vi "ArdnoLoad.vi"(0 "LINX Resource":T1={"IO"=enum."Remote", "Interface"=enum."Serial", "LINX Device Config"={"Interface"=enum."Serial", "COM Port"="COM13", "TCP Configuration"={"IP Address"="", "Port"=0}, "Device Family"=1, "Device ID"=1, "Device Name"="myRIO-1900", "TCP Ref"=refnum, "Channels"={"DI"=[0, 1, 2, 3, 4, 5, 6, 7, 8, 9, 10, 11, 12, 13, 14, 15, 16, 17, 18, 19, 20, 21, 22, 23, 24, 25, 26, 27, 28, 29, 30, 31, 32, 33, 34, 35, 36, 37, 38, 39, 40, 41, 42, 43, 44, 45, 46], "DO"=[0, 1, 2, 3, 4, 5, 6, 7, 8, 9, 10, 11, 12, 13, 14, 15, 16, 17, 18, 19, 20, 21, 22, 23, 24, 25, 26, 27, 28, 29, 30, 31, 32, 33, 34, 35, 36, 37, 38, 39, 40, 41, 42, 43, 44, 45, 46], "AI"=[0, 1, 2, 3, 4, 5, 6, 7, 8, 9, 10, 11], "AO"=[], "PWM"=[3, 5, 6, 9, 10], "QE"=[], "UART"=[0, 1], "I2C 2"=[0], "SPI"=[0], "CAN"=[], "Servo"=[], "AI Ref (V)"=0.0, "AI Resolution (Bits)"=0, "AO Ref (V)"=0.0, "AO Resolution (Bits)"=0}}}, 1 "Single / Multiring?":u16(ring) items=["OneRing", "8-Ring"], 5 "Channel":u32, 7 "Ring":u16, 11 "error in (no error)":errorcluster, 12 "All Rings":bool) -> (4 "LINX Resource out":T1, 14 "ValveStates":bool[](array[boolean]), 15 "error out":errorcluster)   [LabVIEW 2018, in "Arduino.lvlib"]
uses:
  Arduino.lvlib
  <vilib>/MakerHub/LINX/Private/Type Defs/LINX Ref.ctl
  <vilib>/MakerHub/LINX/Private/Type Defs/Platform.ctl
  <vilib>/MakerHub/LINX/Private/Type Defs/Interface.ctl
  <vilib>/MakerHub/LINX/Private/Device/Type Defs/LINX Device Config.ctl
  <vilib>/MakerHub/LINX/Private/Device/Type Defs/TCP Config.ctl
  <vilib>/MakerHub/LINX/Private/Device/Type Defs/Channels.ctl
  <vilib>/MakerHub/LINX/Public/Peripherals/Digital/Digital Write N Chans.vi
  <vilib>/MakerHub/LINX/Private/Local IO/LinxDigitalWrite.vi
  <vilib>/MakerHub/LINX/Public/Utilities/Check Channel.vi
  <vilib>/MakerHub/LINX/Private/Utilties/Generate Error.vi
  <vilib>/MakerHub/LINX/LMH-LINX.lvlib
  <vilib>/MakerHub/LINX/Private/Device/Device.lvlib
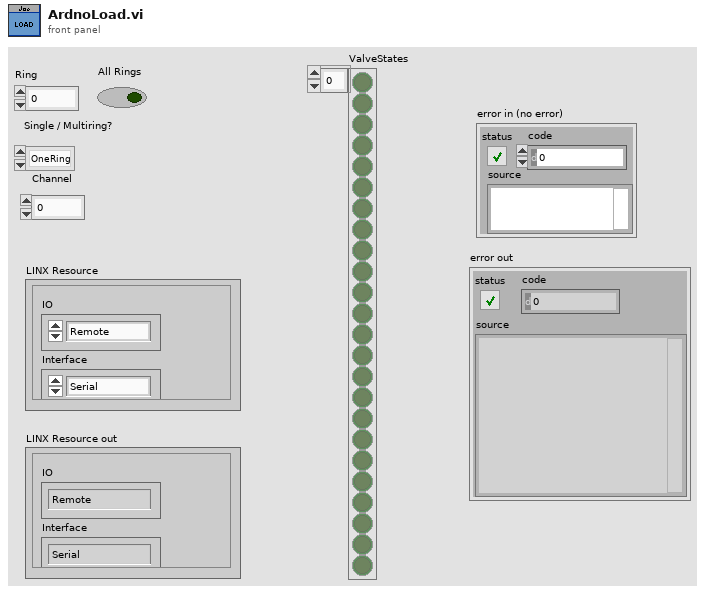
[diagram p1: front panel]
types:
  T1 = typedef "LMH-LINX.lvlib/LINX Ref.ctl" = cluster{"IO":T2, "Interface":T3, "LINX Device Config":T4}
  T2 = typedef "LMH-LINX.lvlib/Platform.ctl" = enum16{"Remote", "Local"}
  T3 = typedef "LMH-LINX.lvlib/Interface.ctl" = enum16{"Serial", "TCP"}
  T4 = typedef "LMH-LINX.lvlib/Device.lvlib/LINX Device Config.ctl" = cluster{"Interface":T3, "COM Port":refnum<visa-resource-name>, "TCP Configuration":T5, "Device Family":u8, "Device ID":u8, "Device Name":string, "TCP Ref":refnum<k5>, "Channels":T6}
  T5 = typedef "LMH-LINX.lvlib/Device.lvlib/TCP Config.ctl" = cluster{"IP Address":string, "Port":u16}
  T6 = typedef "LMH-LINX.lvlib/Channels.ctl" = cluster{"DI":u8[], "DO":u8[], "AI":u8[], "AO":u8[], "PWM":u8[], "QE":u8[], "UART":u8[], "I2C 2":u8[], "SPI":u8[], "CAN":u8[], "Servo":u8[], "AI Ref (V)":dbl, "AI Resolution (Bits)":u8, "AO Ref (V)":dbl, "AO Resolution (Bits)":u8}
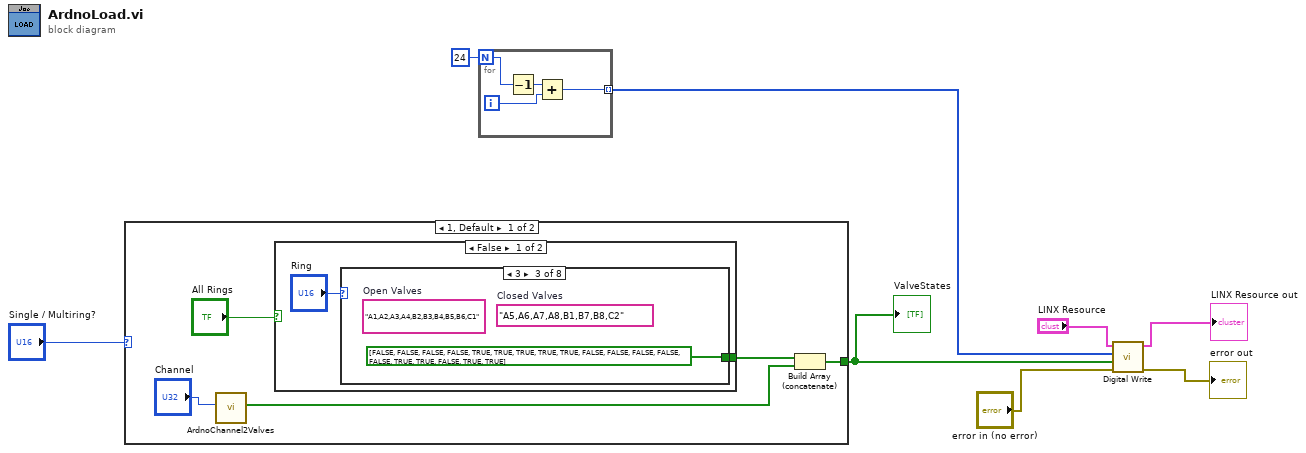
[diagram p0: block diagram]
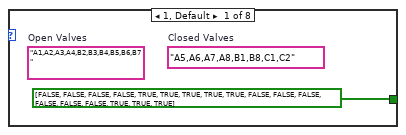
[diagram p2: hidden frame]
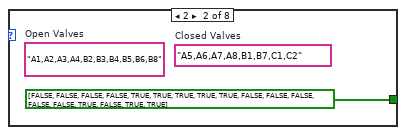
[diagram p3: hidden frame]
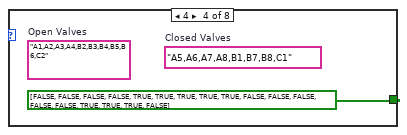
[diagram p4: hidden frame]
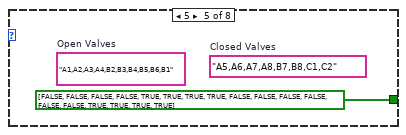
[diagram p5: hidden frame]
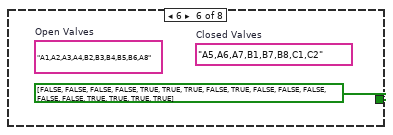
[diagram p6: hidden frame]
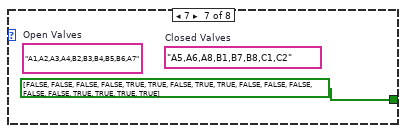
[diagram p7: hidden frame]
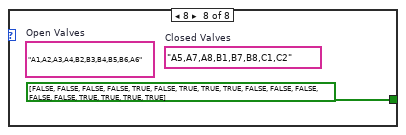
[diagram p8: hidden frame]
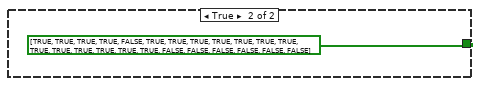
[diagram p9: hidden frame]
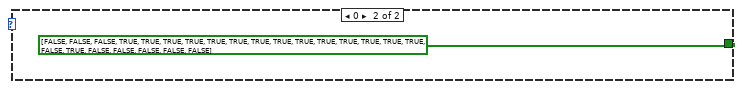
[diagram p10: hidden frame]
diagram:
  n1 = case shown="1, Default" "Single / Multiring?" {
    tunnel: [w9 bool[] [FALSE, FALSE, FALSE, TRUE, TRUE, TRUE, TRUE, TRUE, TRUE, TRUE, TRUE, TRUE, TRUE, TRUE, TRUE, TRUE, TRUE, FALSE, TRUE, FALSE, FALSE, FALSE, FALSE, FALSE]] -> w2
    frame 1, Default {
      n2 = call "ArdnoChannel2Valves.vi"("Channel"="Channel") -> ("Valve State"=w10:bool[])  [unwired: 9 in]
      n3 = case shown="False" "All Rings" {
        tunnel: [w14 bool[] [TRUE, TRUE, TRUE, TRUE, FALSE, TRUE, TRUE, TRUE, TRUE, TRUE, TRUE, TRUE, TRUE, TRUE, TRUE, TRUE, TRUE, TRUE, FALSE, FALSE, FALSE, FALSE, FALSE, FALSE]] -> w11
        frame False {
          n4 = case shown="3" "Ring" {
            tunnel: [bool[] [FALSE, FALSE, FALSE, FALSE, TRUE, TRUE, TRUE, TRUE, TRUE, FALSE, FALSE, FALSE, FALSE, FALSE, FALSE, TRUE, TRUE, TRUE] bool[] [FALSE, FALSE, FALSE, FALSE, TRUE, TRUE, TRUE, TRUE, TRUE, FALSE, FALSE, FALSE, FALSE, FALSE, TRUE, FALSE, TRUE, TRUE] bool[] [FALSE, FALSE, FALSE, FALSE, TRUE, TRUE, TRUE, TRUE, TRUE, FALSE, FALSE, FALSE, FALSE, FALSE, TRUE, TRUE, FALSE, TRUE, TRUE] bool[] [FALSE, FALSE, FALSE, FALSE, TRUE, TRUE, TRUE, TRUE, TRUE, FALSE, FALSE, FALSE, FALSE, FALSE, TRUE, TRUE, TRUE, FALSE] bool[] [FALSE, FALSE, FALSE, FALSE, TRUE, TRUE, TRUE, TRUE, FALSE, FALSE, FALSE, FALSE, FALSE, FALSE, TRUE, TRUE, TRUE, TRUE] bool[] [FALSE, FALSE, FALSE, FALSE, TRUE, TRUE, TRUE, FALSE, TRUE, FALSE, FALSE, FALSE, FALSE, FALSE, TRUE, TRUE, TRUE, TRUE] bool[] [FALSE, FALSE, FALSE, FALSE, TRUE, TRUE, FALSE, TRUE, TRUE, FALSE, FALSE, FALSE, FALSE, FALSE, TRUE, TRUE, TRUE, TRUE] bool[] [FALSE, FALSE, FALSE, FALSE, TRUE, FALSE, TRUE, TRUE, TRUE, FALSE, FALSE, FALSE, FALSE, FALSE, TRUE, TRUE, TRUE, TRUE]] -> w14
            frame 1, Default {
              (unwired) "A5,A6,A7,A8,B1,B8,C1,C2"  # Closed Valves
              (unwired) "A1,A2,A3,A4,B2,B3,B4,B5,B6,B7"  # Open Valves
            }
            frame 2 {
              (unwired) "A5,A6,A7,A8,B1,B7,C1,C2"  # Closed Valves
              (unwired) "A1,A2,A3,A4,B2,B3,B4,B5,B6,B8"  # Open Valves
            }
            frame 3 {
              (unwired) "A5,A6,A7,A8,B1,B7,B8,C2"  # Closed Valves
              (unwired) "A1,A2,A3,A4,B2,B3,B4,B5,B6,C1"  # Open Valves
            }
            frame 4 {
              (unwired) "A5,A6,A7,A8,B1,B7,B8,C1"  # Closed Valves
              (unwired) "A1,A2,A3,A4,B2,B3,B4,B5,B6,C2"  # Open Valves
            }
            frame 5 {
              (unwired) "A5,A6,A7,A8,B7,B8,C1,C2"  # Closed Valves
              (unwired) "A1,A2,A3,A4,B2,B3,B4,B5,B6,B1"  # Open Valves
            }
            frame 6 {
              (unwired) "A5,A6,A7,B1,B7,B8,C1,C2"  # Closed Valves
              (unwired) "A1,A2,A3,A4,B2,B3,B4,B5,B6,A8"  # Open Valves
            }
            frame 7 {
              (unwired) "A5,A6,A8,B1,B7,B8,C1,C2"  # Closed Valves
              (unwired) "A1,A2,A3,A4,B2,B3,B4,B5,B6,A7"  # Open Valves
            }
            frame 8 {
              (unwired) "A5,A7,A8,B1,B7,B8,C1,C2"  # Closed Valves
              (unwired) "A1,A2,A3,A4,B2,B3,B4,B5,B6,A6"  # Open Valves
            }
          }
        }
        frame True {
        }
      }
      n5 = Build Array (concatenate)(w11, w10) -> (w9:bool[])
    }
    frame 0 {
    }
  }
  "ValveStates" <- w2
  n6 = for {
    N: 24 -> [w29]
    tunnel: [w26] -> w3 mode=indexing
    i -> [w27]
    n7 = Decrement(x=w29) -> (x-1=w28:i32)
    n8 = Add(x=w28, y=w27) -> (x+y=w26:i32)
  }
  n9 = call-poly <vilib>:"Digital Write.vi"("Error In"="error in (no error)", "Values"=w2, "DO Channels"=w3, "LINX Resource"="LINX Resource") -> ("Error Out"=→"error out":errorcluster, "LINX Resource"=→"LINX Resource out":T1)  [unwired: 6 in]
